vi "用m-n产生不重复一维数组.vi"(1 "N":dbl, 2 "M":dbl) -> (0 "数组":dbl[](array[numeric]))   [LabVIEW 2009]
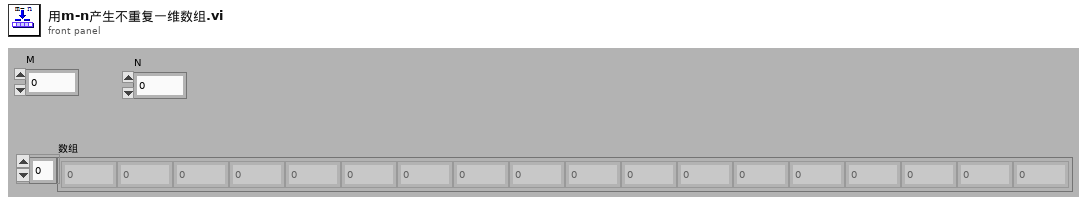
[diagram p1: front panel]
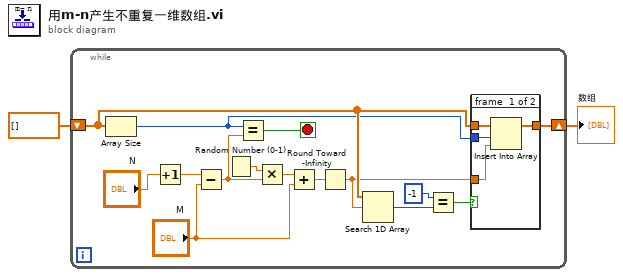
[diagram p0: block diagram]
diagram:
  n1 = while {
    shift-right: [w12] -> w1
    shift-left: dbl[] [] ("数组") -> [w14]
    stop <- w9 stop-if-true
    n2 = Array Size(array=w14) -> (size(s)=w11:i32)
    n3 = Increment(x="N") -> (x+1=w4:dbl)
    n4 = Subtract(x=w4, y="M") -> (x-y=w8:dbl)
    n5 = Random Number (0-1)() -> (number: 0 to 1=w17:dbl)
    n6 = Equal?(x=w11, y=w8) -> (x = y?=w9:bool)
    n7 = Multiply(x=w17, y=w8) -> (x*y=w6:dbl)
    n8 = Add(x=w6, y="M") -> (x+y=w5:dbl)
    n9 = Round Toward -Infinity(1:w5) -> (0:w13:dbl)
    n10 = Search 1D Array(1D array=w14, element=w13) -> (index of element=w16:i32)  [unwired: 1 in]
    n11 = Equal?(x=-1, y=w16) -> (x = y?=w10:bool)
    n12 = case shown="真" w10 {
      tunnel: w14 -> [w21 w22]
      tunnel: w11 -> [w20 _]
      tunnel: w13 -> [w19 _]
      tunnel: [w18 w22] -> w12
      frame #0 {
        n13 = Insert Into Array(array=w21, index=w20, new element=w19) -> (w18:dbl[])
      }
      frame #1 {
      }
    }
  }
  "数组" <- w1
